vi "checkHostAvailable.vi"(0 "HGF_Reference":refnum<class "HGF_Reference.lvclass">, 2 "timeout\n in ms (-1)":i32, 5 "error in (no error)":errorcluster) -> (11 "STOP":bool, 14 "dup HGF_Reference":refnum<class "HGF_Reference.lvclass">, 16 "dup timeout\n in ms (-1)":i32, 19 "error out":errorcluster)   [LabVIEW 2009, in "MoAgSy.lvlib" / "MoAgSy_Host.lvclass"]
doc: "<B>public</B> VI checks if the Host is available. If the Host isn't available for 6 times in a row or an error occurred, stop is true.\n\nF.Berck@gsi.de\nGSI Darmstadt 2009"
uses:
  MoAgSy_Host.lvclass
  HGF_BaseClasses/HGF_Reference/HGF_Reference.lvclass
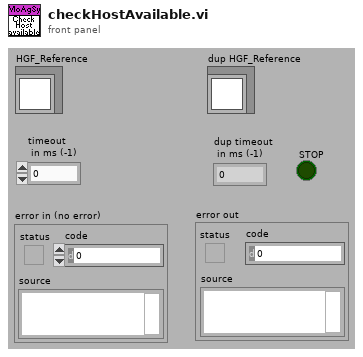
[diagram p1: front panel]
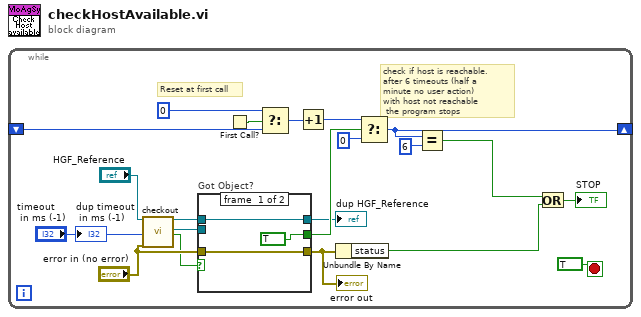
[diagram p0: block diagram]
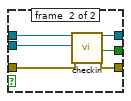
[diagram p2: hidden frame]
diagram:
  n1 = while {
    shift-right: [w7] -> _
    shift-left: _ -> [w5]
    stop <- TRUE stop-if-true
    # "Reset at first call"
    # "check if host is reachable.\nafter 6 timeouts (half a\nminute no user action) \nwith host not reachable\n the program stops"
    n2 = call "checkout.vi"("HGF_Reference"="HGF_Reference", "timeout in ms (-1)"="timeout\n in ms (-1)", "error in (no error)"="error in (no error)") -> ("dup HGF_Reference"=w10:refnum<class "HGF_Reference.lvclass">, "Object"=w11:refnum<class>, "got object?"=w12:bool)  [unwired: 14 out]
    n3 = case "Got Object?" shown="True" w12 {
      tunnel: w10 -> [w22 w30]
      tunnel: w11 -> [_ w29]
      tunnel: "error in (no error)" -> [w24 w28]
      tunnel: [w24 w27] -> w14
      tunnel: [TRUE ("timed out?") w26] -> w17
      tunnel: [w22 w25] -> w1
      frame #0 {
      }
      frame #1 {
        n4 = call "checkin.vi"("HGF_Reference"=w30, "Object"=w29, "error in (no error)"=w28) -> ("dup HGF_Reference"=w25:refnum<class "HGF_Reference.lvclass">, "timed out?"=w26:bool, "error out"=w27:errorcluster)  [unwired: 1 in, 13 out]
      }
    }
    "dup HGF_Reference" <- w1
    "error out" <- w14
    n5 = First Call?() -> (First Call?: T/F=w3:bool)
    n6 = Select(t=0, s=w3, f=w5) -> (s? t:f=w4:i32)
    n7 = Increment(x=w4) -> (x+1=w16:i32)
    n8 = Unbundle By Name(w14) -> ("status"=w15:bool)
    n9 = Select(t=w16, s=w17, f=0) -> (s? t:f=w7:i32)
    n10 = Equal?(x=w7, y=6) -> (x = y?=w20:bool)
    n11 = Or(x=w20, y=w15) -> (x .or. y?=→"STOP":bool)
    "dup timeout\n in ms (-1)" <- "timeout\n in ms (-1)"
  }
